vi "Set Voltage.vi"(6 "wait for reply (T)":bool=TRUE, 8 "error in":errorcluster, 10 "Voltage":dbl, 11 "Module ID":i32=-1) -> (0 "error out":errorcluster, 1 "timed out?":bool, 2 "Command":string)   [LabVIEW 2019, in "Inversor.lvlib"]
doc: "Set Voltage\n\n_____\nCreated using DQMH Framework: Event Scripter 7.1.0.1503."
uses:
  Inversor.lvlib
  Set Voltage Argument--cluster.ctl
  Set Voltage (Reply Payload)--cluster.ctl
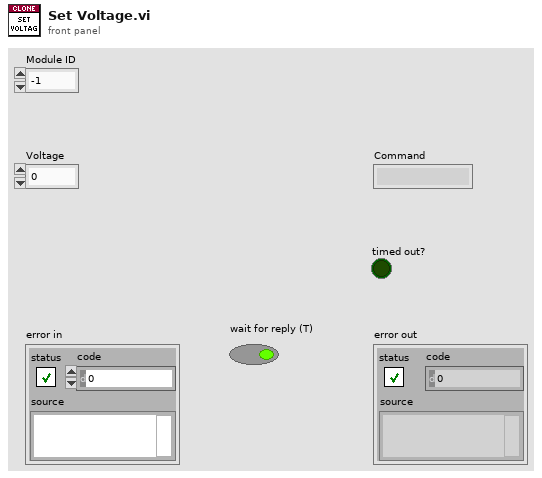
[diagram p1: front panel]
types:
  T1 = typedef "Inversor.lvlib/Set Voltage Argument--cluster.ctl" = cluster{"Module ID":i32, "Voltage":dbl, "Wait Notifier":refnum<notifier>, "wait for reply":bool}
  T2 = typedef "Inversor.lvlib/Request Events--cluster.ctl" = cluster{"Stop Module":refnum<user-event>, "Show Panel":refnum<user-event>, "Hide Panel":refnum<user-event>, "Show Diagram":refnum<user-event>, "Get Module Execution Status":refnum<user-event>, "Local Instance":T3, "Private.Request Privado":refnum<user-event>, "Set Voltage":refnum<user-event>, "Request Simple":refnum<user-event>}
  T3 = typedef "Inversor.lvlib/Local Instance Request Events--cluster.ctl" = cluster{"Request Privado Local":refnum<user-event>}
  T4 = typedef "Inversor.lvlib/Set Voltage (Reply Payload)--cluster.ctl" = cluster{"Module ID":i32, "Command":string, "error":errorcluster, "Response":string}
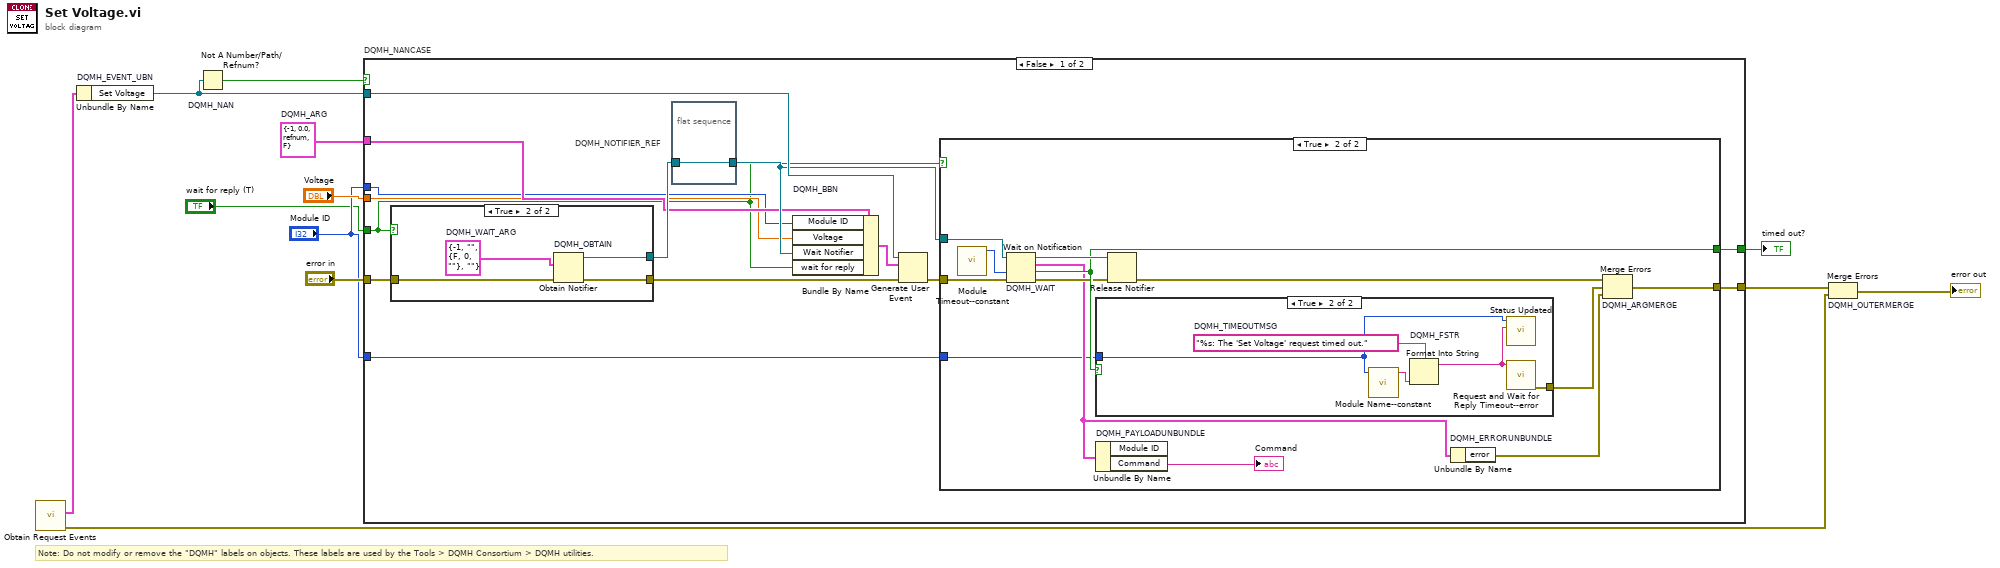
[diagram p0: block diagram]
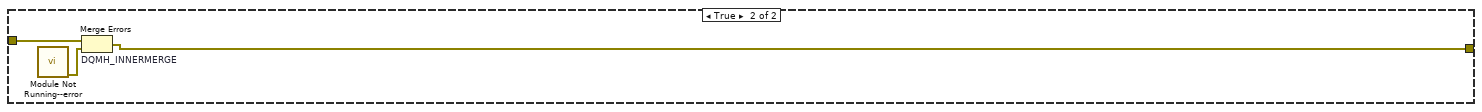
[diagram p5: hidden frame]
diagram:
  w6 = T1 {"Module ID"=-1, "Voltage"=0.0, "Wait Notifier"=refnum, "wait for reply"=FALSE}  # DQMH_ARG
  # "Note: Do not modify or remove the \"DQMH\" labels on objects. These labels are used by the Tools > DQMH Consortium > DQMH utilities."
  n1 = call "Obtain Request Events.vi"() -> ("error out"=w2:errorcluster, "Inversor Request Events"=w1:T2)  [unwired: 10 in]
  n2 = Unbundle By Name "DQMH_EVENT_UBN"(w1) -> ("Set Voltage"=w10:refnum<user-event>)
  n3 = Not A Number/Path/Refnum? "DQMH_NAN"(number/path/refnum=w10) -> (NaN/Path/Refnum?=w9:bool)
  n4 = case "DQMH_NANCASE" shown="False" w9 {
    tunnel: "error in" -> [w26 w54]
    tunnel: w10 -> [w24 _]
    tunnel: [w21 w53] -> w7
    tunnel: [w22 _] -> w8
    tunnel: w6 -> [w17 _]
    tunnel: "Module ID" -> [w16 _]
    tunnel: "Voltage" -> [w15 _]
    tunnel: "Module ID" -> [w14 _]
    tunnel: "wait for reply (T)" -> [w13 _]
    frame False {
      n5 = case shown="True" w13 {
        tunnel: w26 -> [w47 w51]
        tunnel: [w47 w50] -> w23
        tunnel: [_ w48] -> w19
        frame False {
        }
        frame True {
          w49 = T4 {"Module ID"=-1, "Command"="", "error"={"status"=FALSE, "code"=0, "source"=""}, "Response"=""}  # DQMH_WAIT_ARG
          n6 = Obtain Notifier "DQMH_OBTAIN"(notification data type=w49, error in (no error)=w51) -> (notifier out=w48:refnum<notifier>, error out=w50:errorcluster)  [unwired: 2 in, 1 out]
        }
      }
      n7 = flat-sequence "DQMH_NOTIFIER_REF" {
        tunnel: w19 -> [w27]
        tunnel: [w27] -> w18
        frame #0 {
        }
      }
      n8 = Bundle By Name "DQMH_BBN"(cluster=w17, "Module ID"=w16, "Voltage"=w15, "Wait Notifier"=w18, "wait for reply"=w13) -> (w20:T1)
      n9 = Generate User Event(user event=w24, event data cluster=w20, error in=w23) -> (error out=w25:errorcluster)  [unwired: 1 in, 1 out]
      n10 = case shown="True" w13 {
        tunnel: w25 -> [w28 w41]
        tunnel: w18 -> [_ w40]
        tunnel: [_ w38] -> w22
        tunnel: [w28 w37] -> w21
        tunnel: w14 -> [_ w29]
        frame False {
        }
        frame True {
          n11 = call "Module Timeout--constant.vi"() -> ("Module Timeout"=w31:i32)  [unwired: 11 in]
          n12 = Wait on Notification "DQMH_WAIT"(notifier=w40, timeout in ms (-1)=w31, error in (no error)=w41) -> (notifier out=w39:refnum<notifier>, notification=w32:T4, timed out?=w38:bool, error out=w36:errorcluster)  [unwired: 1 in]
          n13 = case shown="True" w38 {
            tunnel: [_ w44] -> w33
            tunnel: w29 -> [_ w42]
            frame False {
            }
            frame True {
              w46 = "%s: The 'Set Voltage' request timed out."  # DQMH_TIMEOUTMSG
              n14 = call "Module Name--constant.vi"("Module ID"=w42) -> ("Module Name"=w43:string)  [unwired: 10 in]
              n15 = Format Into String "DQMH_FSTR"(format string=w46, w43) -> (resulting string=w45:string)  [unwired: 2 in, 1 out]
              n16 = call "Status Updated.vi"("Status"=w45, "Module ID"=w42) -> ()  [unwired: 9 in, 1 out]
              n17 = call "Request and Wait for Reply Timeout--error.vi"("Error Message"=w45) -> ("error out"=w44:errorcluster)  [unwired: 10 in]
            }
          }
          n18 = Unbundle By Name "DQMH_PAYLOADUNBUNDLE"(w32) -> ("Command"=→"Command":string)  [unwired: 1 out]
          n19 = Release Notifier(notifier=w39, error in (no error)=w36) -> (error out=w35:errorcluster)  [unwired: 1 in, 2 out]
          n20 = Unbundle By Name "DQMH_ERRORUNBUNDLE"(w32) -> ("error"=w34:errorcluster)
          n21 = Merge Errors "DQMH_ARGMERGE"(w35, w33, w34) -> (w37:errorcluster)
        }
      }
    }
    frame True {
      n22 = call "Module Not Running--error.vi"() -> ("error out"=w52:errorcluster)  [unwired: 11 in]
      n23 = Merge Errors "DQMH_INNERMERGE"(w54, w52) -> (w53:errorcluster)
    }
  }
  "timed out?" <- w8
  n24 = Merge Errors "DQMH_OUTERMERGE"(w7, w2) -> (→"error out":errorcluster)
